vi "link -- read For_RPR file.vi"(8 "rus out file path":path=path "C:/Data/GloveBox/Pu/rprcyl") -> (0 "freqs":dbl[](array[numeric]))   [LabVIEW 2014]
uses:
  <vilib>/Utility/file.llb/Read From Spreadsheet File (string).vi
panel:
  in  "Color Box":u32(colorbox)
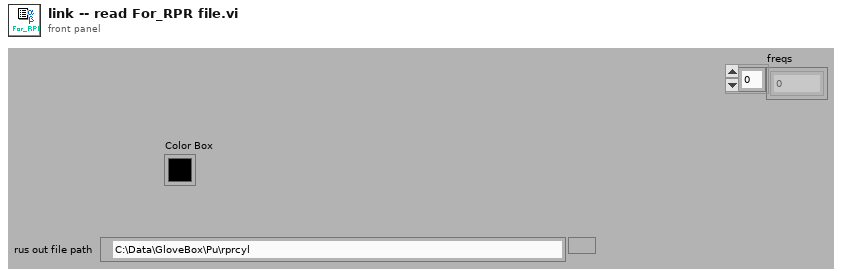
[diagram p1: front panel]
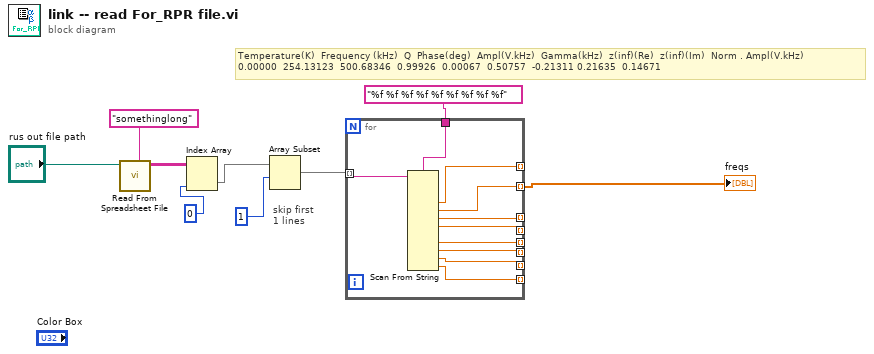
[diagram p0: block diagram]
diagram:
  # "Temperature(K)\t\tFrequency (kHz)\t\tQ\t\tPhase(deg)\t\tAmpl(V.kHz)\t\tGamma(kHz)\t\tz(inf)(Re)\t\tz(inf)(Im)\t\tNorm . Ampl(V.kHz)\n0.00000\t\t254.13123\t\t500.68346\t\t0.99926\t\t0.00067\t\t0.50757\t\t-0.21311\t0.21635\t\t0.14671"
  # "skip first \n1 lines"
  n1 = call-poly <vilib>:"Read From Spreadsheet File.vi"("delimiter (\\t)"="somethinglong" ("delimiter (\\t)"), "file path (dialog if empty)"="rus out file path") -> ("all rows"=w5:string[][])  [unwired: 5 in, 4 out]
  n2 = Index Array(array=w5, index (col)=0 ("index (row)")) -> (element=w6:string[])  [unwired: 1 in]
  n3 = Array Subset(array=w6, index=1 ("index (row)")) -> (w4:string[])  [unwired: 1 in]
  n4 = for {
    tunnel: w4 -> [w19] mode=indexing
    tunnel: [w18] -> _ mode=indexing
    tunnel: [w17] -> w2 mode=indexing
    tunnel: [w16] -> _ mode=indexing
    tunnel: "%f %f %f %f %f %f %f %f %f" ("format string") -> [w15]
    tunnel: [w14] -> _ mode=indexing
    tunnel: [w13] -> _ mode=indexing
    tunnel: [w12] -> _ mode=indexing
    tunnel: [w11] -> _ mode=indexing
    tunnel: [w10] -> _ mode=indexing
    n5 = Scan From String(format string=w15, input string=w19) -> (output 1=w18:dbl, output 2=w17:dbl, output 3=w16:dbl, output 4=w14:dbl, output 6=w13:dbl, output 7=w12:dbl, output 8=w11:dbl, output 9=w10:dbl)  [unwired: 12 in, 3 out]
  }
  "freqs" <- w2
